vi "StationMeteo.vi"() -> ()   [LabVIEW 2018]
uses:
  <vilib>/Instr/_visa.llb/VISA Configure Serial Port (Instr).vi
panel:
  out "Chaîne":string
  in  "stop":bool
  in  "Nom de ressource VISA":refnum<visa-resource-name>
  # "1. Brancher la carte Arduino sur un port USB\n2. Choisir le port COM de la carte dans la liste déroulante \"Nom de ressource VISA\"\n3. Lancer le programme"
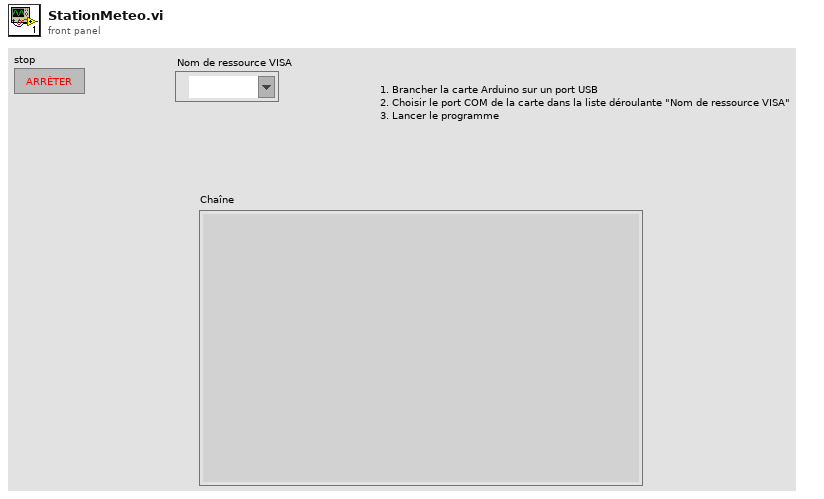
[diagram p1: front panel]
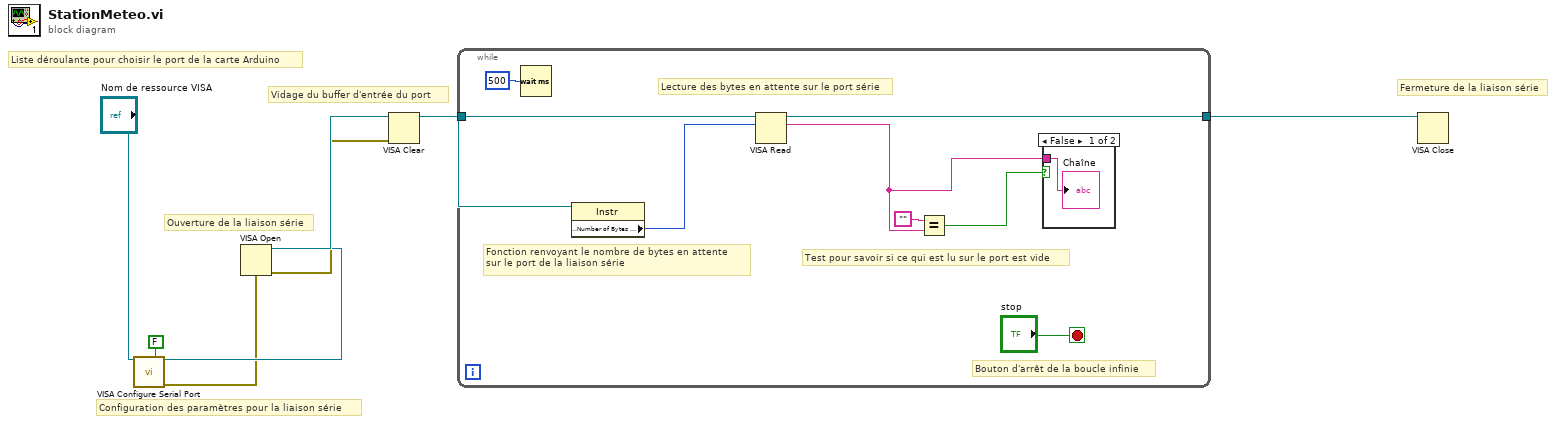
[diagram p0: block diagram]
diagram:
  # "Vidage du buffer d'entrée du port"
  # "Ouverture de la liaison série"
  # "Configuration des paramètres pour la liaison série"
  # "Liste déroulante pour choisir le port de la carte Arduino"
  # "Fermeture de la liaison série"
  n1 = call-poly "VISA Configure Serial Port"("VISA resource name"="Nom de ressource VISA", "Enable Termination\nChar (T)"=FALSE ("Enable Termination\nChar (T)")) -> ("VISA resource name out"=w5:refnum<visa-resource-name>, "error out"=w3:errorcluster)  [unwired: 12 in]
  n2 = VISA Open(error in (no error)=w3, VISA resource name=w5) -> (VISA resource name=w7:refnum<visa-resource-name>, error out=w2:errorcluster)  [unwired: 3 in]
  n3 = VISA Clear(VISA resource name=w7, error in (no error)=w2) -> (VISA resource name out=w6:refnum<visa-resource-name>)  [unwired: 1 out]
  n4 = while {
    tunnel: w6 -> [w15]
    tunnel: [w13] -> w1
    stop <- "stop" stop-if-true
    # "Lecture des bytes en attente sur le port série"
    # "Fonction renvoyant le nombre de bytes en attente\nsur le port de la liaison série"
    # "Test pour savoir si ce qui est lu sur le port est vide"
    # "Bouton d'arrêt de la boucle infinie"
    n5 = Wait (ms)(milliseconds to wait=u32 500 ("attente (ms)")) -> ()  [unwired: 1 out]
    n6 = property class="Instr"(reference=w15) -> ("Serial Settings:Number of Bytes at Serial Port"=w14:u32)  [unwired: 1 in, 2 out]
    n7 = VISA Read(VISA resource name=w15, byte count=w14) -> (VISA resource name out=w13:refnum<visa-resource-name>, read buffer=w9:string)  [unwired: 1 in, 2 out]
    n8 = Equal?(x="", y=w9) -> (x = y?=w10:bool)
    n9 = case shown="False" w10 {
      tunnel: w9 -> [w17 _]
      frame False {
        "Chaîne" <- w17
      }
      frame True {
      }
    }
  }
  n10 = VISA Close(VISA resource name=w1) -> ()  [unwired: 1 in, 1 out]
